vi "Server Data FGV.vi"(8 "error in (no error)":errorcluster, 10 "Action":enum16{"Initialize", "Check", "Close"}(ring)=enum."Check") -> (0 "error out":errorcluster, 1 "Responses Ref":refnum<data-value>, 3 "Request Queue":refnum<queue>, 4 "Server Running":bool)   [LabVIEW 2017, in "JSONRPC Server.lvclass"]
uses:
  JSONRPC Server.lvclass
  Request/Request.lvclass
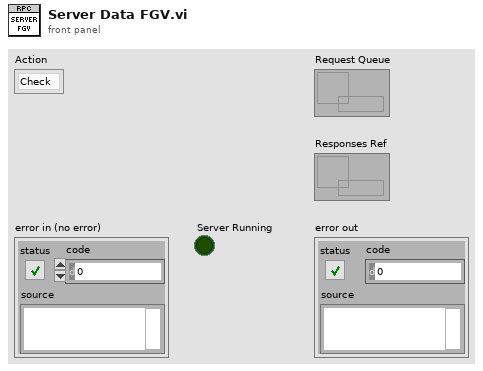
[diagram p1: front panel]
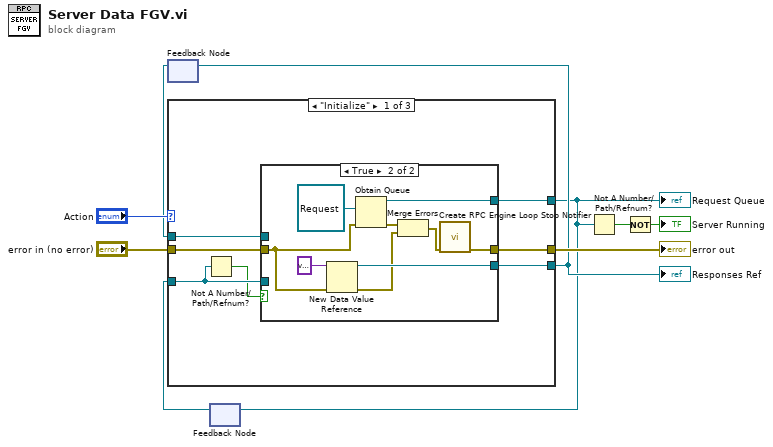
[diagram p0: block diagram]
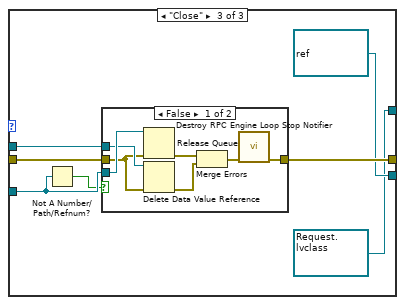
[diagram p4: hidden frame]
diagram:
  n1 = feedback #1() -> (w4:refnum<data-value>)  [unwired: 1 in]
  n2 = feedback #2() -> (w8:refnum<queue>)  [unwired: 1 in]
  n3 = case shown="\"Initialize\"" "Action" {
    tunnel: [w16 w30 refnum<queue> refnum ("queue out")] -> w3
    tunnel: w8 -> [w11 w30 w33]
    tunnel: "error in (no error)" -> [w15 w31 w36]
    tunnel: [w14 w31 w38] -> w6
    tunnel: [w13 w29 refnum<data-value> refnum ("data value reference")] -> w5
    tunnel: w4 -> [w12 w29 w37]
    frame "Initialize" {
      n4 = Not A Number/Path/Refnum?(number/path/refnum=w11) -> (NaN/Path/Refnum?=w10:bool)
      n5 = case shown="True" w10 {
        tunnel: [w18 w28] -> w16
        tunnel: w15 -> [w19 w21]
        tunnel: [w19 w20] -> w14
        tunnel: w11 -> [w18 _]
        tunnel: [w17 w23] -> w13
        tunnel: w12 -> [w17 _]
        frame False {
        }
        frame True {
          n6 = New Data Value Reference(data value=variant, error in=w21) -> (data value reference=w23:refnum<data-value>, error out=w22:errorcluster)
          n7 = Obtain Queue(element data type=refnum<class "Request.lvclass"> refnum ("Request.lvclass"), error in (no error)=w21) -> (queue out=w28:refnum<queue>, error out=w26:errorcluster)  [unwired: 3 in, 1 out]
          n8 = Merge Errors(w26, w22) -> (w25:errorcluster)
          n9 = call "Create RPC Engine Loop Stop Notifier.vi"("error in (no error)"=w25) -> ("error out"=w20:errorcluster)  [unwired: 10 in]
        }
      }
    }
    frame "Check" {
    }
    frame "Close" {
      n10 = Not A Number/Path/Refnum?(number/path/refnum=w33) -> (NaN/Path/Refnum?=w32:bool)
      n11 = case shown="False" w32 {
        tunnel: w33 -> [w45 _]
        tunnel: [w39 w46] -> w38
        tunnel: w37 -> [w43 _]
        tunnel: w36 -> [w41 w46]
        frame False {
          n12 = Release Queue(queue=w45, error in (no error)=w41) -> (error out=w44:errorcluster)  [unwired: 1 in, 2 out]
          n13 = Delete Data Value Reference(data value reference=w43, error in=w41) -> (error out=w42:errorcluster)  [unwired: 1 out]
          n14 = Merge Errors(w44, w42) -> (w40:errorcluster)
          n15 = call "Destroy RPC Engine Loop Stop Notifier.vi"("error in (no error)"=w40) -> ("error out"=w39:errorcluster)  [unwired: 10 in]
        }
        frame True {
        }
      }
    }
  }
  "error out" <- w6
  "Request Queue" <- w3
  "Responses Ref" <- w5
  n16 = feedback-in #1(w5) -> ()
  n17 = feedback-in #2(w3) -> ()
  n18 = Not A Number/Path/Refnum?(number/path/refnum=w3) -> (NaN/Path/Refnum?=w2:bool)
  n19 = Not(x=w2) -> (.not. x?=→"Server Running":bool)
